vi "TestQbusLogger1.vi"   [LabVIEW 2014]
uses:
  <vilib>/addons/Qbus/Qbus.lvclass
  <vilib>/addons/InsightCM/Devices/Shared/QbusHelpers/QbusHelper.lvlib
  <vilib>/addons/TraceLogger/TraceLogger.lvlib
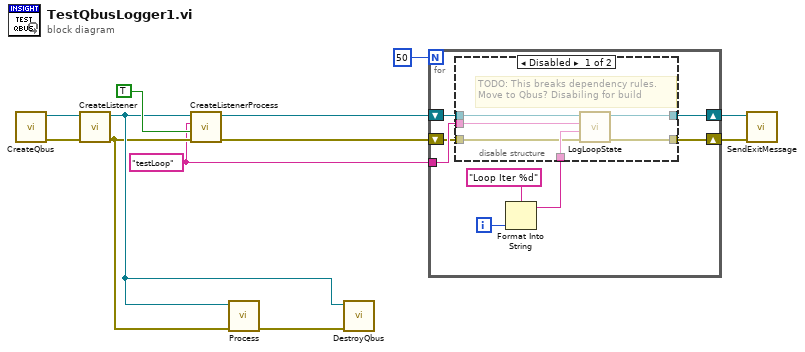
[diagram p0: block diagram]
diagram:
  w1 = "testLoop" ("ProcessName")
  n1 = call <vilib>:"CreateQbus.vi"() -> ("error out"=w6:errorcluster, "Qbus"=w7:refnum<class "Qbus.lvclass">)  [unwired: 10 in]
  n2 = call <vilib>:"CreateListener.vi"("error in (no error)"=w6, "qbus in"=w7) -> ("error out"=w4:errorcluster, "qbus out"=w5:refnum<class "Qbus.lvclass">)  [unwired: 8 in]
  n3 = call <vilib>:"CreateListenerProcess.vi"("error in (no error)"=w4, "master"=TRUE ("Master"), "process name"=w1, "Qbus in"=w5) -> ("error in (no error)"=w2:errorcluster, "Qbus out"=w3:refnum<class "Qbus.lvclass">)  [unwired: 6 in]
  n4 = call <vilib>:"Process.vi"("error in (no error)"=w4, "qbus in"=w5) -> ("error out"=w9:errorcluster)  [unwired: 9 in]
  n5 = call <vilib>:"DestroyQbus.vi"("error in (no error)"=w9, "Qbus"=w5) -> ()  [unwired: 9 in, 1 out]
  n6 = for {
    N: 50 -> [_]
    tunnel: w1 -> [w16]
    shift-right: [w15] -> w11
    shift-left: w3 -> [w20]
    shift-right: [w13] -> w10
    shift-left: w2 -> [w14]
    i -> [w18]
    n7 = Format Into String(format string="Loop Iter %d", w18) -> (resulting string=w17:string)  [unwired: 2 in, 1 out]
    n8 = disable-structure shown="Disabled" {
      disable-tunnel: w20 -> [w26 _]
      disable-tunnel: w17 -> [w25 _]
      disable-tunnel: w16 -> [w24 _]
      disable-tunnel: [w23 _] -> w15
      disable-tunnel: w14 -> [w22 _]
      disable-tunnel: [w21 _] -> w13
      frame Disabled {
        # "TODO: This breaks dependency rules.\nMove to Qbus? Disabiling for build"
        n9 = call <vilib>:"LogLoopState.vi"("error in (no error)"=w22, "loop action"=w25, "process name"=w24, "Qbus in"=w26) -> ("error out"=w21:errorcluster, "Qbus out"=w23:refnum<class "Qbus.lvclass">)  [unwired: 6 in]
      }
      frame Enabled {
      }
    }
  }
  n10 = call <vilib>:"SendExitMessage.vi"("error in (no error)"=w10, "Qbus in"=w11) -> ()  [unwired: 8 in, 2 out]
